vi "DAQ_Output_Task.vi"(8 "error in":errorcluster) -> (0 "error out":errorcluster, 3 "task out":refnum<k21>)   [LabVIEW 2015]
uses:
  <vilib>/DAQmx/create/channels.llb/DAQmx Create Channel (AO-Voltage-Basic).vi
  <vilib>/DAQmx/create/channels.llb/DAQmx Create Channel (AO-Current-Basic).vi
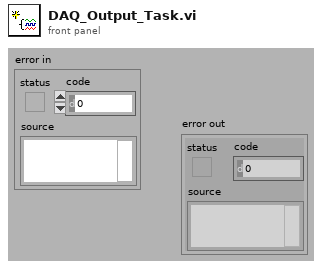
[diagram p1: front panel]
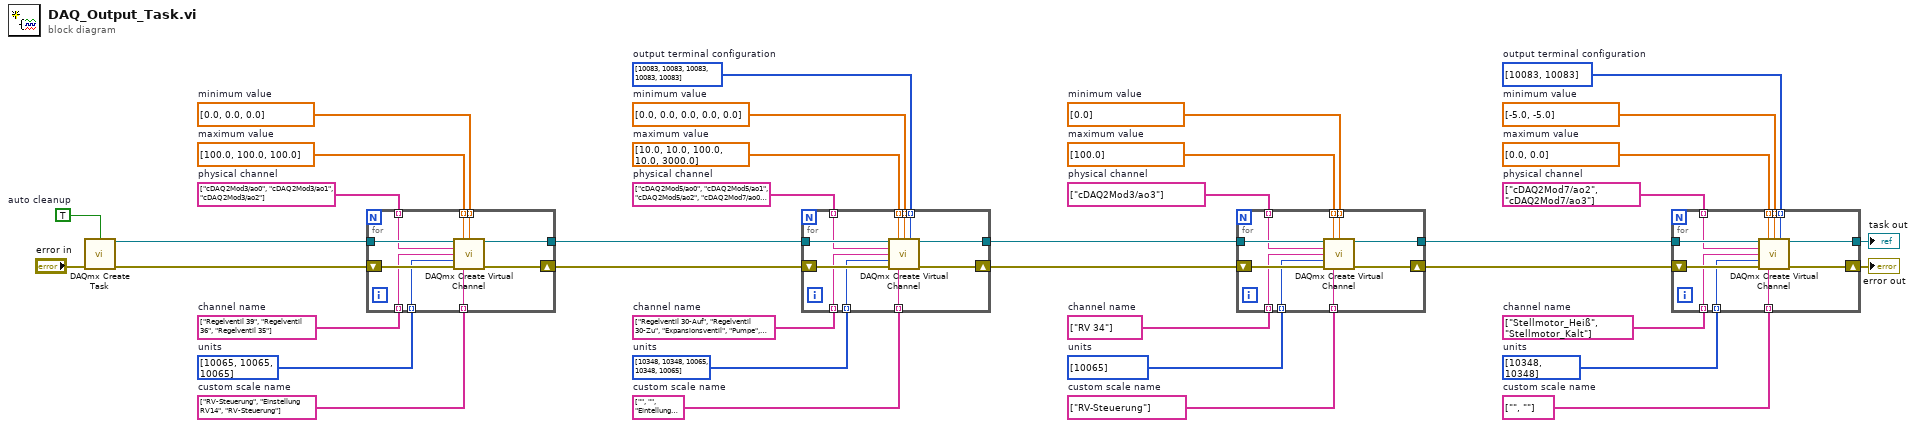
[diagram p0: block diagram]
diagram:
  w1 = i32[] [10083, 10083] items=["Default"=-1, "RSE"=10083, "Differential"=10106, "Pseudodifferential"=12529]  # output terminal configuration
  w7 = string[] ["", ""]  # custom scale name
  w6 = i32[] [10348, 10348] items=["Volts"=10348, "From Custom Scale"=10065]  # units
  w5 = string[] ["Stellmotor_Heiß", "Stellmotor_Kalt"]  # channel name
  w4 = string[] ["cDAQ2Mod7/ao2", "cDAQ2Mod7/ao3"]  # physical channel
  w8 = dbl[] [0.0, 0.0]  # maximum value
  w9 = dbl[] [-5.0, -5.0]  # minimum value
  w15 = string[] ["RV-Steuerung"]  # custom scale name
  w14 = i32[] [10065] items=["Amps"=10342, "From Custom Scale"=10065]  # units
  w13 = string[] ["RV 34"]  # channel name
  w12 = string[] ["cDAQ2Mod3/ao3"]  # physical channel
  w16 = dbl[] [100.0]  # maximum value
  w17 = dbl[] [0.0]  # minimum value
  w19 = i32[] [10083, 10083, 10083, 10083, 10083] items=["Default"=-1, "RSE"=10083, "Differential"=10106, "Pseudodifferential"=12529]  # output terminal configuration
  w24 = string[] ["", "", "Eintellung ExpV", "", "Verdichter_UPM"]  # custom scale name
  w23 = i32[] [10348, 10348, 10065, 10348, 10065] items=["Volts"=10348, "From Custom Scale"=10065]  # units
  w22 = string[] ["Regelventil 30-Auf", "Regelventil 30-Zu", "Expansionsventil", "Pumpe", "Verdichter"]  # channel name
  w21 = string[] ["cDAQ2Mod5/ao0", "cDAQ2Mod5/ao1", "cDAQ2Mod5/ao2", "cDAQ2Mod7/ao0", "cDAQ2Mod7/ao1"]  # physical channel
  w25 = dbl[] [10.0, 10.0, 100.0, 10.0, 3000.0]  # maximum value
  w26 = dbl[] [0.0, 0.0, 0.0, 0.0, 0.0]  # minimum value
  w32 = string[] ["RV-Steuerung", "Einstellung RV14", "RV-Steuerung"]  # custom scale name
  w31 = i32[] [10065, 10065, 10065] items=["Amps"=10342, "From Custom Scale"=10065]  # units
  w30 = string[] ["Regelventil 39", "Regelventil 36", "Regelventil 35"]  # channel name
  w29 = string[] ["cDAQ2Mod3/ao0", "cDAQ2Mod3/ao1", "cDAQ2Mod3/ao2"]  # physical channel
  w33 = dbl[] [100.0, 100.0, 100.0]  # maximum value
  w34 = dbl[] [0.0, 0.0, 0.0]  # minimum value
  w36 = TRUE  # auto cleanup
  n1 = call <vilib>:"DAQmx Create Task.vi"("auto cleanup"=w36, "error in"="error in") -> ("task out"=w35:refnum<k21>, "error out"=w37:errorcluster)  [unwired: 12 in]
  n2 = for {
    tunnel: w35 -> [w46]
    tunnel: w34 -> [w47] mode=indexing
    tunnel: w33 -> [w48] mode=indexing
    tunnel: w32 -> [w39] mode=indexing
    tunnel: w31 -> [w40] mode=indexing
    tunnel: w30 -> [w42] mode=indexing
    tunnel: w29 -> [w41] mode=indexing
    tunnel: [w44] -> w27
    shift-right: [w43] -> w28
    shift-left: w37 -> [w45]
    n3 = call-poly <vilib>:"DAQmx Create Virtual Channel.vi"("task in"=w46, "maximum value"=w48, "minimum value"=w47, "physical channels"=w41, "name to assign"=w42, "units"=w40, "error in"=w45, "custom scale name"=w39) -> ("task out"=w44:refnum<k21>, "error out"=w43:errorcluster)  [unwired: 6 in]
  }
  n4 = for {
    tunnel: w27 -> [w57]
    tunnel: w26 -> [w58] mode=indexing
    tunnel: w25 -> [w59] mode=indexing
    tunnel: w24 -> [w50] mode=indexing
    tunnel: w23 -> [w51] mode=indexing
    tunnel: w22 -> [w53] mode=indexing
    tunnel: w21 -> [w52] mode=indexing
    tunnel: [w55] -> w18
    shift-right: [w54] -> w20
    shift-left: w28 -> [w56]
    tunnel: w19 -> [w49] mode=indexing
    n5 = call-poly <vilib>:"DAQmx Create Virtual Channel.vi"("task in"=w57, "maximum value"=w59, "minimum value"=w58, "output terminal configuration"=w49, "physical channels"=w52, "name to assign"=w53, "units"=w51, "error in"=w56, "custom scale name"=w50) -> ("task out"=w55:refnum<k21>, "error out"=w54:errorcluster)  [unwired: 5 in]
  }
  n6 = for {
    tunnel: w18 -> [w67]
    tunnel: w17 -> [w68] mode=indexing
    tunnel: w16 -> [w69] mode=indexing
    tunnel: w15 -> [w60] mode=indexing
    tunnel: w14 -> [w61] mode=indexing
    tunnel: w13 -> [w63] mode=indexing
    tunnel: w12 -> [w62] mode=indexing
    tunnel: [w65] -> w10
    shift-right: [w64] -> w11
    shift-left: w20 -> [w66]
    n7 = call-poly <vilib>:"DAQmx Create Virtual Channel.vi"("task in"=w67, "maximum value"=w69, "minimum value"=w68, "physical channels"=w62, "name to assign"=w63, "units"=w61, "error in"=w66, "custom scale name"=w60) -> ("task out"=w65:refnum<k21>, "error out"=w64:errorcluster)  [unwired: 6 in]
  }
  n8 = for {
    tunnel: w10 -> [w78]
    tunnel: w9 -> [w79] mode=indexing
    tunnel: w8 -> [w80] mode=indexing
    tunnel: w7 -> [w71] mode=indexing
    tunnel: w6 -> [w72] mode=indexing
    tunnel: w5 -> [w74] mode=indexing
    tunnel: w4 -> [w73] mode=indexing
    tunnel: [w76] -> w3
    shift-right: [w75] -> w2
    shift-left: w11 -> [w77]
    tunnel: w1 -> [w70] mode=indexing
    n9 = call-poly <vilib>:"DAQmx Create Virtual Channel.vi"("task in"=w78, "maximum value"=w80, "minimum value"=w79, "output terminal configuration"=w70, "physical channels"=w73, "name to assign"=w74, "units"=w72, "error in"=w77, "custom scale name"=w71) -> ("task out"=w76:refnum<k21>, "error out"=w75:errorcluster)  [unwired: 5 in]
  }
  "error out" <- w2
  "task out" <- w3
